vi "ModeMgr.Get Mode.vi"(8 "error in (no error)":errorcluster, 11 "ModeMgr In":refnum<class "Mode Manager.lvclass">) -> (0 "error out":errorcluster, 1 "Settings":T1[](array[typedef]), 2 "Mode":string, 3 "ModeMgr Out":refnum<class "Mode Manager.lvclass">)   [LabVIEW 2018, in "Mode Manager.lvclass"]
uses:
  Mode Manager.lvclass
  ModeMgr.Mode Settings.ctl
  Mode Manager.lvclass/Mode Manager.ctl
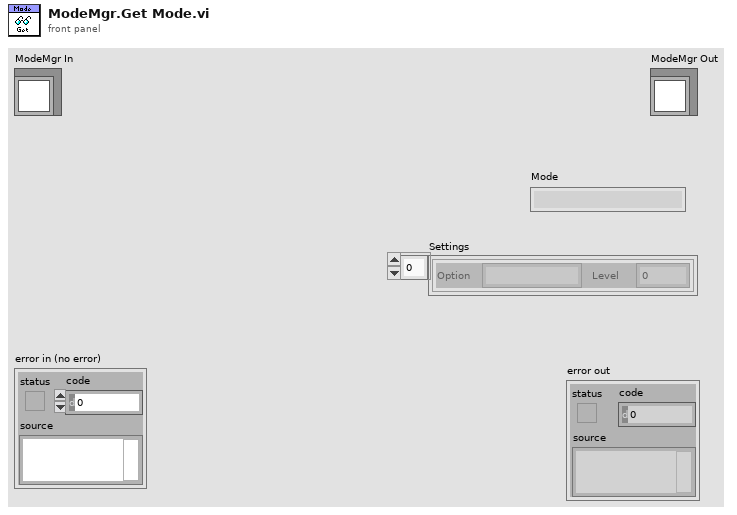
[diagram p1: front panel]
types:
  T1 = typedef "ModeMgr.Mode Settings.ctl" = cluster{"Option":string, "Level":i32}
  T2 = typedef "ModeMgr.ModeConfig.ctl" = cluster{"Name":string, "Color":string, "Settings":T1[], "Password":string}
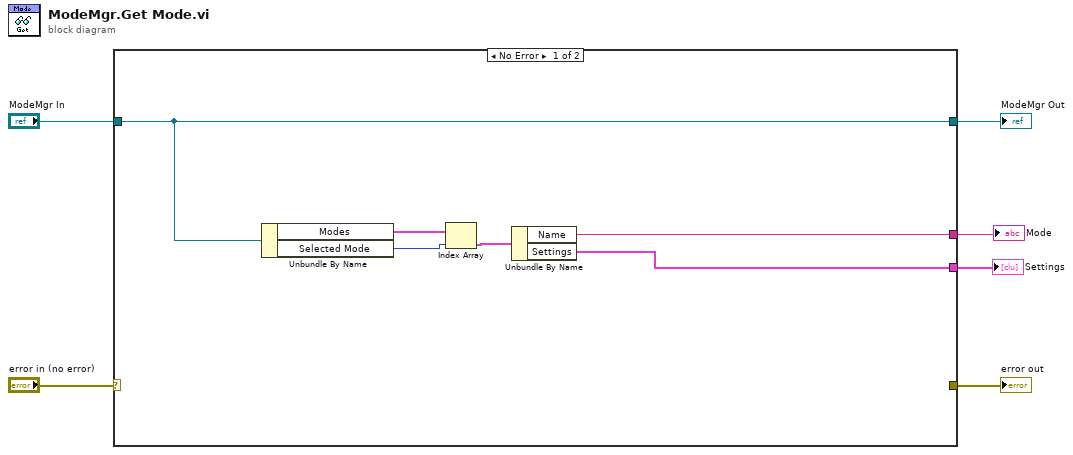
[diagram p0: block diagram]
diagram:
  n1 = case shown="No Error" "error in (no error)" {
    selector: "error in (no error)" -> [_ w14]
    tunnel: [_ w14] -> w5
    tunnel: [w12 w13] -> w3
    tunnel: "ModeMgr In" -> [w12 w13]
    tunnel: [w8 _] -> w2
    tunnel: [w7 _] -> w1
    frame No Error {
      n2 = Unbundle By Name(w12) -> ("Modes"=w11:T2[], "Selected Mode"=w9:i32)
      n3 = Index Array(array=w11, index=w9) -> (element=w10:T2)
      n4 = Unbundle By Name(w10) -> ("Name"=w8:string, "Settings"=w7:T1[])
    }
    frame Error {
    }
  }
  "error out" <- w5
  "ModeMgr Out" <- w3
  "Settings" <- w1
  "Mode" <- w2
